vi "ThermalCam.vi"() -> ()   [LabVIEW 2024, in "ThermalCam ISGPlugin.lvlib"]
uses:
  ThermalCam ISGPlugin.lvlib
  CTI/Identity.ctl
  <vilib>/Plug-In SDKs/InstrumentStudio/Plugin Events Enum.ctl
  CTI/GPIO Pull.ctl
  1e6ec9c9-fb05-4fd0-b05f-9caec19ae962.vi
  8524c294-126d-4a78-a4f4-5e8209367d85.vi
  7e432e81-cfec-40ee-91ac-c41f46aea1a5.vi
  81a0c2b0-cfce-4e0a-bc55-b9605872672a.vi
  913d5d43-3022-4ea6-842c-e3943c591263.vi
  <extravilib>/ChannelInstances/Tag-bool/Instantiate.vi
  <extravilib>/ChannelInstances/Tag-bool/EndpointRead.vi
  <extravilib>/ChannelInstances/Tag-bool/Endpoint.vi
  <vilib>/gmath/interp.llb/Interpolate 2D (2d X,Y).vi
  CTI/Session/Session.lvclass
  <vilib>/gmath/NI_Gmath.lvlib
  <vilib>/ptbypt/NI_PtbyPt.lvlib
  <extravilib>/ChannelInstances/Tag-bool.lvlib
  CTI/VisaComms/VisaComms.lvclass
  CTI/CTI.lvlib
  <vilib>/Plug-In SDKs/InstrumentStudio/Plugin Session.lvclass
  <vilib>/Plug-In SDKs/InstrumentStudio/InstrumentStudio Plugin SDK.lvlib
panel:
  out "error out 2":errorcluster
  in  "Session Id":u64
  out "Interpolated Frame":dbl[][](graph)
  out "Unprocessed Pixels":dbl[][](graph)
  out "Processing Performance":dbl(graph)=0.0211100999986229
  out "Color Box":u32(colorbox)
  in  "Map selector":T1(ring)=enum."rainbow"
  in  "Pause":bool
  in  "Run Stop":bool
  in  "MICRO-CONTROLLER COM PORT":refnum<visa-resource-name>
  in  "SMOOTHING TYPE":i32(ring)=3 items=["nearest", "bilinear", "bicubic", "bicubic spline"]
  in  "TEMPERATURE RANGE":dbl=12.0
  in  "Interpolate":bool=TRUE
  in  "Max hold":bool
  in  "COMPRESSION":dbl=3.0
  in  "Auto Z Scale":bool=TRUE
  out "AVERAGE MAX":dbl=82.15301832388433 format="%.1f"
  out "Current Max":dbl=82.15301832388433 format="%.1f"
  in  "SMOOTHING ALPHA":dbl=0.4 min=0.0 max=1.0 step=0.05 format="%#_13g"
  out "ON-BOARD TEMP":dbl
  out "FRAME COUNT":i32
  out "Identity 2":T2
  out "error out":errorcluster
  # "ADVANCED PRESENCE SENSOR"
  # "RP2040 + AMG8833 + LabVIEW CTI"
  # "DUT Control Settings"
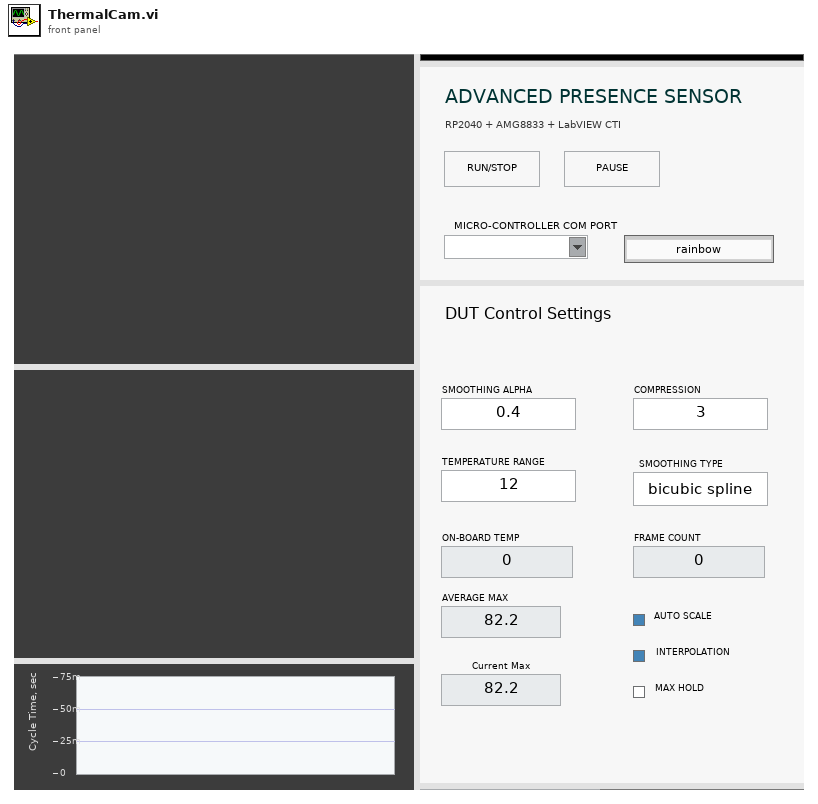
[diagram p1: front panel]
types:
  T1 = enum16{"fire", "rainbow", "grey", "inverse grey", "ice", "original"}
  T2 = typedef "CTI.lvlib/Identity.ctl" = cluster{"Vendor":string, "Model":string, "Serial":string, "Version":string}
  T3 = typedef "InstrumentStudio Plugin SDK.lvlib/Plugin Events Enum.ctl" = enum32{"Shutdown", "Project Saved", "Stop All Outputs", "Generic Message", "Active Pin Map Changed", "Selected Sites Changed"}
  T4 = typedef "Tag-bool.lvlib/))Channel.ctl" = refnum<queue>
  T5 = typedef "CTI.lvlib/GPIO Pull.ctl" = enum16{"None", "Up", "Down", "Both"}
  T6 = typedef "InstrumentStudio Plugin SDK.lvlib/Event Registration Refnum.ctl" = refnum<event-registration>
  T7 = enum16{"No Scaling", "Scale All Objects", "Scale Single Object"}
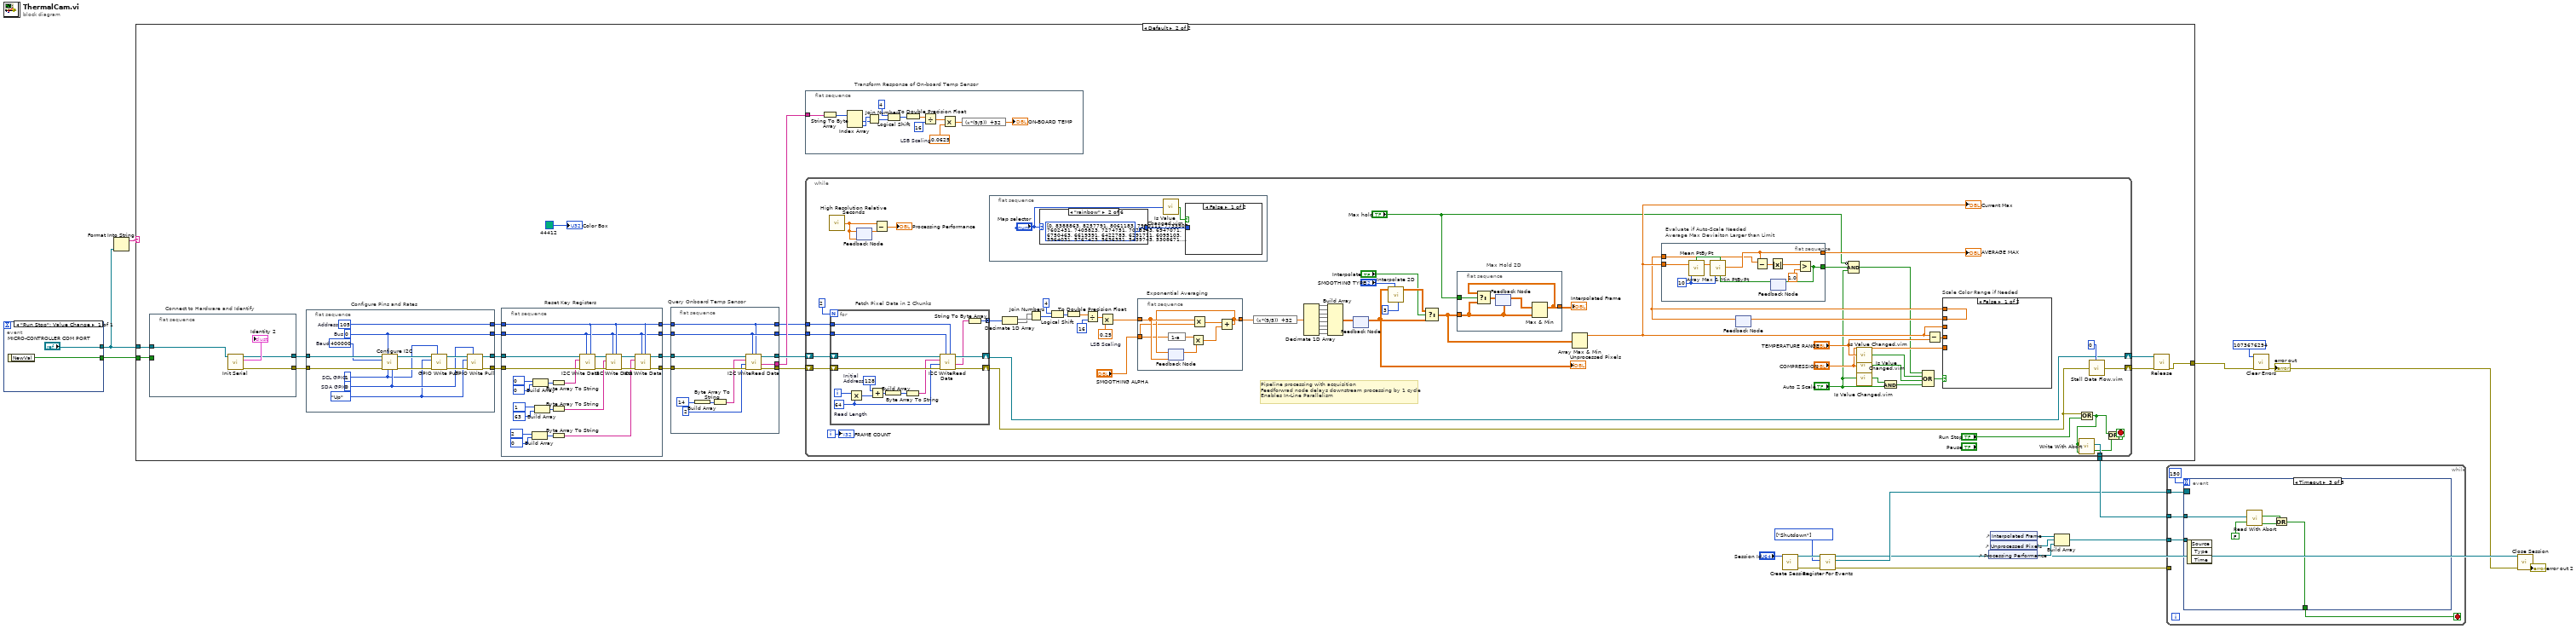
[diagram p0: block diagram]
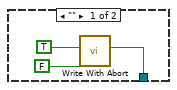
[diagram p2: hidden frame]
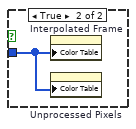
[diagram p3: hidden frame]
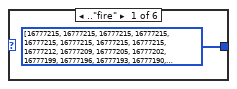
[diagram p4: hidden frame]
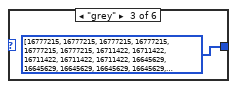
[diagram p5: hidden frame]
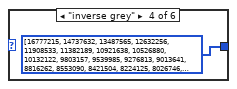
[diagram p6: hidden frame]
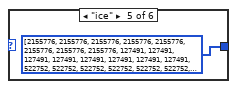
[diagram p7: hidden frame]
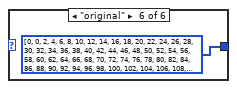
[diagram p8: hidden frame]
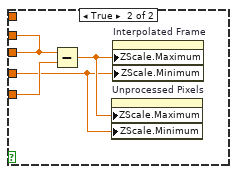
[diagram p9: hidden frame]
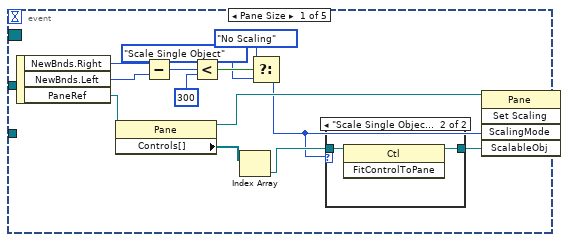
[diagram p10: hidden frame]
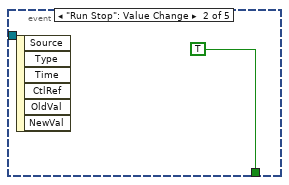
[diagram p12: hidden frame]
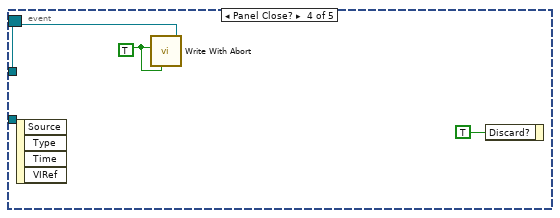
[diagram p13: hidden frame]
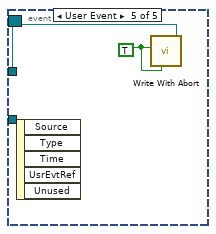
[diagram p14: hidden frame]
diagram:
  w10 = T3[] [enum."Shutdown"] items=["Shutdown", "Project Saved", "Stop All Outputs", "Generic Message", "Active Pin Map Changed", "Selected Sites Changed"] ("Events To Register")
  n1 = event shown="[0] \"Run Stop\": Value Change" {
    selector: _ -> [_]
    dyn-events: _ -> [_]
    timeout: _ -> [_]
    tunnel: [w21] -> w4
    tunnel: ["MICRO-CONTROLLER COM PORT"] -> w3
    event "Run Stop": Value Change {
      n2 = event-data() -> ("NewVal"=w21:bool)  [unwired: 1 in]
    }
  }
  n3 = Format Into String(w3) -> (resulting string=w2:string)  [unwired: 3 in, 1 out]
  n4 = case shown="Default" w2 {
    tunnel: [w24 w31] -> w14
    tunnel: w4 -> [_ w29]
    tunnel: w3 -> [_ w28]
    tunnel: [_ w25] -> w1
    frame "" {
      n5 = call <extravilib>:"Write With Abort.vi"("abort"=FALSE, "element"=TRUE) -> ("channel"=w24:T4)  [unwired: 7 in, 2 out]
    }
    frame Default {
      n6 = flat-sequence "Connect to Hardware and Identify" {
        tunnel: [w109] -> w46
        tunnel: [w108] -> w45
        tunnel: w29 -> [_]
        tunnel: w28 -> [w107]
        frame #0 {
          n7 = call "Init Serial.vi"("VISA resource name in"=w107) -> ("error out"=w108:errorcluster, "Identity"=→"Identity 2":T2, "Session"=w109:refnum<class "Session.lvclass">)  [unwired: 8 in]
        }
      }
      n8 = flat-sequence "Configure Pins and Rates" {
        tunnel: w46 -> [w106]
        tunnel: w45 -> [w105]
        tunnel: [w99] -> w44
        tunnel: [w98] -> w43
        tunnel: [w97] -> w38
        tunnel: [w96] -> w37
        frame #0 {
          w93 = GPIO_Pull."Up" ("GPIO Pull")
          w96 = u8 105  # Address
          w97 = u8 0  # Bus
          w94 = 1  # SCL GPIO
          w95 = 0  # SDA GPIO
          w104 = u32 400000  # Baud
          n9 = call "Configure I2C.vi"("SDA GPIO"=w95, "SCL GPIO"=w94, "I2C #"=w97, "error in (no error)"=w105, "Baud"=w104, "Session in"=w106) -> ("error out"=w102:errorcluster, "Session out"=w103:refnum<class "Session.lvclass">)  [unwired: 4 in]
          n10 = call "GPIO Write Pull.vi"("GPIO #"=w94, "error in (no error)"=w102, "GPIO Pull"=w93, "Session in"=w103) -> ("error out"=w100:errorcluster, "Session out"=w101:refnum<class "Session.lvclass">)  [unwired: 6 in]
          n11 = call "GPIO Write Pull.vi"("GPIO #"=w95, "error in (no error)"=w100, "GPIO Pull"=w93, "Session in"=w101) -> ("error out"=w99:errorcluster, "Session out"=w98:refnum<class "Session.lvclass">)  [unwired: 6 in]
        }
      }
      n12 = flat-sequence "Reset Key Registers" {
        tunnel: w44 -> [w92]
        tunnel: w43 -> [w91]
        tunnel: [w79] -> w42
        tunnel: [w73] -> w40
        tunnel: w38 -> [w71]
        tunnel: w37 -> [w72]
        tunnel: [w72] -> w35
        tunnel: [w71] -> w34
        frame #0 {
          n13 = Build Array(u8 2 ("Address"), u8 0 ("Address")) -> (w75:u8[])
          n14 = Build Array(u8 0 ("Address"), u8 0 ("Address")) -> (w87:u8[])
          n15 = Build Array(u8 1 ("Address"), u8 63 ("Address")) -> (w83:u8[])
          n16 = Byte Array To String(unsigned byte array=w87) -> (string=w90:string)
          n17 = Byte Array To String(unsigned byte array=w83) -> (string=w80:string)
          n18 = Byte Array To String(unsigned byte array=w75) -> (string=w74:string)
          n19 = call "I2C Write Data.vi"("Address"=w72, "I2C #"=w71, "error in (no error)"=w92, "Data"=w90, "Session in"=w91) -> ("error out"=w86:errorcluster, "Session out"=w84:refnum<class "Session.lvclass">)  [unwired: 5 in]
          n20 = call "I2C Write Data.vi"("Address"=w72, "I2C #"=w71, "error in (no error)"=w86, "Data"=w80, "Session in"=w84) -> ("error out"=w85:errorcluster, "Session out"=w78:refnum<class "Session.lvclass">)  [unwired: 5 in]
          n21 = call "I2C Write Data.vi"("Address"=w72, "I2C #"=w71, "error in (no error)"=w85, "Data"=w74, "Session in"=w78) -> ("error out"=w79:errorcluster, "Session out"=w73:refnum<class "Session.lvclass">)  [unwired: 5 in]
        }
      }
      n22 = flat-sequence "Query Onboard Temp Sensor" {
        tunnel: w42 -> [w57]
        tunnel: [w56] -> w41
        tunnel: w40 -> [w55]
        tunnel: [w54] -> w39
        tunnel: w34 -> [w48]
        tunnel: w35 -> [w47]
        tunnel: [w50] -> w36
        tunnel: [w48] -> w33
        tunnel: [w47] -> w32
        frame #0 {
          n23 = Build Array(u8 14 ("Address")) -> (w52:u8[])
          n24 = Byte Array To String(unsigned byte array=w52) -> (string=w51:string)
          n25 = call "I2C WriteRead Data.vi"("Address"=w47, "I2C #"=w48, "error in (no error)"=w57, "Len"=u8 2 ("Read Len"), "Write Data"=w51, "Session in"=w55) -> ("error out"=w56:errorcluster, "Read Data"=w50:string, "Session out"=w54:refnum<class "Session.lvclass">)  [unwired: 3 in]
        }
      }
      n26 = while {
        tunnel: w33 -> [w161]
        tunnel: w32 -> [w160]
        shift-right: [w117] -> w27
        shift-left: w41 -> [w163]
        shift-right: [w111] -> w26
        shift-left: w39 -> [w162]
        tunnel: [w116] -> w31
        i -> [w159]
        stop <- w114 stop-if-true
        w147 = 0.25  # LSB Scaling
        # "Pipeline processing with acquisition\nFeedforwrad node delays downstream processing by 1 cycle\nEnables In-Line Parallelism"
        n27 = call <vilib>:"High Resolution Relative Seconds.vi"() -> ("relative seconds"=w151:dbl)
        n28 = for "Fetch Pixel Data in 2 Chunks" {
          N: 2 -> [_]
          shift-right: [w217] -> w124
          shift-left: w163 -> [w218]
          shift-right: [w216] -> w111
          shift-left: w162 -> [w219]
          tunnel: w161 -> [w215]
          tunnel: w160 -> [w214]
          tunnel: [w220] -> w174 mode=concatenating
          i -> [w209]
          w210 = u8 64  # Read Length
          w211 = u8 128  # Initial Address
          n29 = Multiply(x=w209, y=w210) -> (x*y=w207:i32)
          n30 = Add(x=w211, y=w207) -> (x+y=w208:i32)
          n31 = Build Array(w208) -> (w221:i32[])
          n32 = Byte Array To String(unsigned byte array=w221) -> (string=w213:string)
          n33 = call "I2C WriteRead Data.vi"("Address"=w214, "I2C #"=w215, "error in (no error)"=w218, "Len"=w210, "Write Data"=w213, "Session in"=w219) -> ("error out"=w217:errorcluster, "Read Data"=w212:string, "Session out"=w216:refnum<class "Session.lvclass">)  [unwired: 3 in]
          n34 = String To Byte Array(string=w212) -> (unsigned byte array=w220:u8[])
        }
        n35 = feedback-in #1(w151) -> ()
        n36 = feedback #1(w151) -> (w150:dbl)
        n37 = Subtract(x=w151, y=w150) -> (x-y=→"Processing Performance":dbl)
        n38 = flat-sequence {
          frame #0 {
            n39 = case shown="\"rainbow\"" "Map selector" {
              tunnel: [u32[] [16777215, 16777215, 16777215, 16777215, 16777215, 16777215, 16777215, 16777215, 16777212, 16777209, 16777205, 16777202, 16777199, 16777196, 16777193, 16777190, 16777186, 16777183, 16777180, 16777177, 16777174, 16777170, 16777167, 16777164, 16777161, 16777158, 16777154, 16777151, 16777148, 16777145, 16777142, 16777139, 16777135, 16777132, 16777129, 16777126, 16777123, 16777119, 16777116, 16777113, 16777110, 16777107, 16777103, 16777100, 16777097, 16777094, 16777091, 16777088, 16777084, 16777081, 16777078, 16777075, 16777072, 16777068, 16777065, 16777062, 16777059, 16777056, 16777052, 16777049, 16777046, 16777043, 16777040, 16777037, 16777033, 16777030, 16777027, 16777024, 16777021, 16777017, 16777014, 16777011, 16777008, 16777005, 16777001, 16776998, 16776995, 16776992, 16776989, 16776986, 16776982, 16776979, 16776976, 16776973, 16776970, 16776966, 16776963, 16776960, 16776192, 16775424, 16774400, 16773632, 16772864, 16772096, 16771328, 16770560, 16769536, 16768768, 16768000, 16767232, 16766464, 16765440, 16764672, 16763904, 16763136, 16762368, 16761344, 16760576, 16759808, 16759040, 16758272, 16757504, 16756480, 16755712, 16754944, 16754176, 16753408, 16752384, 16751616, 16750848, 16750080, 16749312, 16748288, 16747520, 16746752, 16745984, 16745216, 16744448, 16743424, 16742656, 16741888, 16741120, 16740352, 16739328, 16738560, 16737792, 16737024, 16736256, 16735232, 16734464, 16733696, 16732928, 16732160, 16731392, 16730368, 16729600, 16728832, 16728064, 16727296, 16726272, 16725504, 16724736, 16723968, 16723200, 16722176, 16721408, 16720640, 16719872, 16719104, 16718336, 16717312, 16716544, 16715776, 16715008, 16714240, 16713216, 16712448, 16711680, 16515072, 16318464, 16056320, 15859712, 15663104, 15466496, 15269888, 15073280, 14811136, 14614528, 14417920, 14221312, 14024704, 13762560, 13565952, 13369344, 13172736, 12976128, 12713984, 12517376, 12320768, 12124160, 11927552, 11730944, 11468800, 11272192, 11075584, 10878976, 10682368, 10420224, 10223616, 10027008, 9830400, 9633792, 9371648, 9175040, 8978432, 8781824, 8585216, 8388608, 8126464, 7929856, 7733248, 7536640, 7340032, 7077888, 6881280, 6684672, 6488064, 6291456, 6029312, 5832704, 5636096, 5439488, 5242880, 5046272, 4784128, 4587520, 4390912, 4194304, 3997696, 3735552, 3538944, 3342336, 3145728, 2949120, 2686976, 2490368, 2293760, 2097152, 1900544, 1703936, 1441792, 1245184, 1048576, 851968, 655360, 393216, 196608, 65793, 65793, 65793, 65793, 65793, 65793, 65793, 65793, 0] ("256 fire") u32[] [0, 8388863, 8257791, 8061183, 7930111, 7733503, 7602431, 7405823, 7274751, 7078143, 6947071, 6750463, 6619391, 6422783, 6291711, 6095103, 5964031, 5767423, 5636351, 5439743, 5308671, 5112063, 4980991, 4784383, 4653311, 4456703, 4325631, 4129023, 3932415, 3801343, 3604735, 3473663, 3277055, 3145983, 2949375, 2818303, 2621695, 2490623, 2294015, 2162943, 1966335, 1835263, 1638655, 1507583, 1310975, 1179903, 983295, 852223, 655615, 524543, 327935, 196863, 511, 1791, 3071, 4351, 5631, 6911, 8191, 9471, 10751, 12031, 13311, 14591, 15871, 17151, 18431, 19711, 20991, 22271, 23551, 24831, 26111, 27391, 28671, 29951, 31231, 32511, 33791, 35071, 36351, 37631, 38911, 40191, 41471, 42751, 44031, 45311, 46591, 47871, 49151, 50431, 51711, 52991, 54271, 55551, 56831, 58111, 59391, 60671, 61951, 63231, 64511, 65532, 65527, 65522, 65517, 65512, 65507, 65502, 65497, 65492, 65487, 65482, 65477, 65472, 65467, 65462, 65457, 65452, 65447, 65442, 65437, 65432, 65427, 65422, 65417, 65412, 65407, 65402, 65397, 65392, 65387, 65382, 65377, 65372, 65367, 65362, 65357, 65352, 65347, 65342, 65337, 65332, 65327, 65322, 65317, 65312, 65307, 65302, 65297, 65292, 65287, 65282, 261888, 589568, 917248, 1244928, 1572608, 1900288, 2227968, 2555648, 2883328, 3211008, 3538688, 3866368, 4194048, 4521728, 4849408, 5177088, 5504768, 5832448, 6160128, 6487808, 6815488, 7143168, 7470848, 7798528, 8126208, 8453888, 8781568, 9109248, 9436928, 9764608, 10092288, 10419968, 10747648, 11075328, 11403008, 11730688, 12058368, 12386048, 12713728, 13041408, 13369088, 13696768, 14024448, 14352128, 14679808, 15007488, 15335168, 15662848, 15990528, 16318208, 16645888, 16775936, 16774656, 16773376, 16772096, 16770816, 16769536, 16768256, 16766976, 16765696, 16764416, 16763136, 16761856, 16760576, 16759296, 16758016, 16756736, 16755456, 16754176, 16752896, 16751616, 16750336, 16749056, 16747776, 16746496, 16745216, 16743936, 16742656, 16741376, 16740096, 16738816, 16737536, 16736256, 16734976, 16733696, 16732416, 16731136, 16729856, 16728576, 16727296, 16726016, 16724736, 16723456, 16722176, 16720896, 16719616, 16718336, 16717056, 16715776, 16714496, 16713216, 16711680] ("rainbow") u32[] [16777215, 16777215, 16777215, 16777215, 16777215, 16777215, 16711422, 16711422, 16711422, 16711422, 16711422, 16645629, 16645629, 16645629, 16645629, 16645629, 16645629, 16579836, 16579836, 16579836, 16579836, 16579836, 16514043, 16514043, 16514043, 16514043, 16514043, 16448250, 16448250, 16448250, 16448250, 16448250, 16316664, 16382457, 16382457, 16382457, 16382457, 16316664, 16316664, 16316664, 16316664, 16250871, 16250871, 16250871, 16250871, 16250871, 16185078, 16185078, 16185078, 16185078, 16119285, 16119285, 16119285, 16119285, 16119285, 16053492, 16053492, 16053492, 16053492, 15987699, 15987699, 15987699, 15987699, 15921906, 15987699, 15921906, 15921906, 15856113, 15856113, 15856113, 15856113, 15856113, 15790320, 15790320, 15790320, 15724527, 15724527, 15724527, 15724527, 15658734, 15658734, 15658734, 15658734, 15592941, 15592941, 15592941, 15592941, 15527148, 15527148, 15527148, 15461355, 15461355, 15461355, 15461355, 15395562, 15395562, 15395562, 15395562, 15329769, 15329769, 15329769, 15263976, 15263976, 15263976, 15198183, 15198183, 15198183, 15198183, 15132390, 15132390, 15132390, 15066597, 15066597, 15066597, 15000804, 15000804, 15000804, 14935011, 14935011, 14935011, 14869218, 14869218, 14869218, 14803425, 14803425, 14803425, 14737632, 14737632, 14671839, 14671839, 14671839, 14606046, 14606046, 14606046, 14540253, 14540253, 14540253, 14474460, 14474460, 14408667, 14408667, 14408667, 14342874, 14342874, 14277081, 14277081, 14277081, 14211288, 14211288, 14145495, 14145495, 14079702, 14079702, 14013909, 14013909, 14013909, 13948116, 13948116, 13882323, 13882323, 13816530, 13816530, 13750737, 13750737, 13684944, 13684944, 13619151, 13619151, 13553358, 13553358, 13487565, 13487565, 13421772, 13421772, 13355979, 13290186, 13290186, 13224393, 13224393, 13158600, 13092807, 13092807, 13027014, 13027014, 12961221, 12895428, 12895428, 12829635, 12763842, 12763842, 12698049, 12632256, 12566463, 12566463, 12500670, 12434877, 12434877, 12369084, 12303291, 12237498, 12171705, 12171705, 12105912, 12040119, 11974326, 11908533, 11842740, 11776947, 11711154, 11645361, 11579568, 11513775, 11447982, 11382189, 11316396, 11250603, 11184810, 11119017, 10987431, 10921638, 10855845, 10790052, 10658466, 10592673, 10461087, 10395294, 10329501, 10197915, 10066329, 10000536, 9868950, 9737364, 9605778, 9474192, 9342606, 9211020, 9079434, 8882055, 8750469, 8553090, 8421504, 8224125, 7960953, 7763574, 7500402, 7237230, 6974058, 6645093, 6316128, 5855577, 5395026, 4868682, 4210752, 3289650, 2105376, 0] ("256 log up") u32[] [16777215, 14737632, 13487565, 12632256, 11908533, 11382189, 10921638, 10526880, 10132122, 9803157, 9539985, 9276813, 9013641, 8816262, 8553090, 8421504, 8224125, 8026746, 7895160, 7697781, 7566195, 7434609, 7303023, 7171437, 7039851, 6908265, 6776679, 6710886, 6579300, 6447714, 6381921, 6316128, 6184542, 6118749, 5987163, 5921370, 5855577, 5789784, 5658198, 5592405, 5526612, 5460819, 5395026, 5329233, 5263440, 5197647, 5131854, 5066061, 5000268, 4934475, 4868682, 4802889, 4737096, 4671303, 4605510, 4605510, 4539717, 4473924, 4408131, 4342338, 4342338, 4276545, 4210752, 4210752, 4144959, 4079166, 4013373, 4013373, 3947580, 3881787, 3881787, 3815994, 3750201, 3750201, 3684408, 3684408, 3618615, 3552822, 3552822, 3487029, 3487029, 3421236, 3421236, 3355443, 3289650, 3289650, 3223857, 3223857, 3158064, 3158064, 3092271, 3092271, 3026478, 3026478, 2960685, 2960685, 2894892, 2894892, 2829099, 2829099, 2763306, 2763306, 2763306, 2697513, 2697513, 2631720, 2631720, 2565927, 2565927, 2500134, 2500134, 2500134, 2434341, 2434341, 2368548, 2368548, 2368548, 2302755, 2302755, 2236962, 2236962, 2236962, 2171169, 2171169, 2171169, 2105376, 2105376, 2105376, 2039583, 2039583, 1973790, 1973790, 1973790, 1907997, 1907997, 1907997, 1842204, 1842204, 1842204, 1776411, 1776411, 1776411, 1710618, 1710618, 1710618, 1644825, 1644825, 1644825, 1579032, 1579032, 1579032, 1579032, 1513239, 1513239, 1513239, 1447446, 1447446, 1447446, 1381653, 1381653, 1381653, 1381653, 1315860, 1315860, 1315860, 1315860, 1250067, 1250067, 1250067, 1184274, 1184274, 1184274, 1184274, 1118481, 1118481, 1118481, 1118481, 1052688, 1052688, 1052688, 1052688, 986895, 986895, 986895, 921102, 921102, 921102, 921102, 921102, 855309, 855309, 855309, 855309, 789516, 789516, 789516, 789516, 723723, 723723, 723723, 723723, 657930, 657930, 657930, 657930, 657930, 592137, 592137, 592137, 592137, 526344, 526344, 526344, 526344, 526344, 460551, 460551, 460551, 460551, 460551, 394758, 394758, 394758, 394758, 328965, 328965, 328965, 328965, 328965, 263172, 263172, 263172, 263172, 263172, 197379, 197379, 197379, 197379, 197379, 131586, 131586, 131586, 131586, 131586, 131586, 65793, 65793, 65793, 65793, 65793, 0, 0, 0, 0, 0, 0] ("256 log down") u32[] [2155776, 2155776, 2155776, 2155776, 2155776, 2155776, 2155776, 2155776, 127491, 127491, 127491, 127491, 127491, 127491, 127491, 127491, 522752, 522752, 522752, 522752, 522752, 522752, 522752, 522752, 64018, 64018, 64018, 64018, 64018, 64018, 64018, 64018, 63778, 63778, 63778, 63778, 63778, 63778, 63778, 63778, 63790, 63790, 63790, 63790, 63790, 63790, 63790, 63790, 63797, 63797, 63797, 63797, 63797, 63797, 63797, 63797, 63807, 63807, 63807, 63807, 63807, 63807, 63807, 63807, 64068, 64068, 64068, 64068, 64068, 64068, 64068, 64068, 63828, 63828, 63828, 63828, 63828, 63828, 63828, 63828, 63833, 63833, 63833, 63833, 63833, 63833, 63833, 63833, 63836, 63836, 63836, 63836, 63836, 63836, 63836, 63836, 63836, 63836, 63836, 63836, 63836, 63836, 63836, 63836, 61790, 61790, 61790, 61790, 61790, 61790, 61790, 61790, 58464, 58464, 58464, 58464, 58464, 58464, 58464, 58464, 55387, 55387, 55387, 55387, 55387, 55387, 55387, 55387, 51286, 51286, 51286, 51286, 51286, 51286, 51286, 51286, 47440, 47440, 47440, 47440, 47440, 47440, 47440, 47440, 40284, 40284, 40284, 40284, 40284, 40284, 40284, 40284, 34154, 34154, 34154, 34154, 34154, 34154, 34154, 34154, 28540, 28540, 28540, 28540, 28540, 28540, 28540, 28540, 20113, 20113, 20113, 20113, 20113, 20113, 20113, 20113, 12193, 12193, 12193, 12193, 12193, 12193, 12193, 12193, 12714, 12714, 12714, 12714, 12714, 12714, 12714, 12714, 7351, 7351, 7351, 7351, 7351, 7351, 7351, 7351, 4800, 4800, 4800, 4800, 4800, 4800, 4800, 4800, 195, 195, 195, 195, 195, 195, 195, 195, 189, 189, 189, 189, 189, 189, 189, 189, 183, 183, 183, 183, 183, 183, 183, 183, 175, 175, 175, 175, 175, 175, 175, 175, 164, 164, 164, 164, 164, 164, 164, 164, 155, 155, 155, 155, 155, 155, 155, 155] ("32 ice") u32[] [0, 0, 2, 4, 6, 8, 10, 12, 14, 16, 18, 20, 22, 24, 26, 28, 30, 32, 34, 36, 38, 40, 42, 44, 46, 48, 50, 52, 54, 56, 58, 60, 62, 64, 66, 68, 70, 72, 74, 76, 78, 80, 82, 84, 86, 88, 90, 92, 94, 96, 98, 100, 102, 104, 106, 108, 110, 112, 114, 116, 118, 120, 122, 124, 126, 128, 130, 132, 134, 136, 138, 140, 142, 144, 146, 148, 150, 152, 154, 156, 158, 160, 162, 164, 166, 168, 170, 172, 174, 176, 178, 180, 182, 184, 186, 188, 190, 192, 194, 196, 198, 200, 202, 204, 206, 208, 210, 212, 214, 216, 218, 220, 222, 224, 226, 228, 230, 232, 234, 236, 238, 240, 242, 244, 246, 248, 250, 252, 255, 131839, 263423, 395007, 526591, 658175, 789759, 921343, 1052927, 1184511, 1316095, 1447679, 1579263, 1710847, 1842431, 1974015, 2105599, 2237183, 2368767, 2500351, 2631935, 2763519, 2895103, 3026687, 3158271, 3289855, 3421439, 3553023, 3684607, 3816191, 3947775, 4079359, 4210943, 4342527, 4474111, 4605695, 4737279, 4868863, 5000447, 5132031, 5263615, 5395199, 5526783, 5658367, 5789951, 5921535, 6053119, 6184703, 6316287, 6447871, 6579455, 6711039, 6842623, 6974207, 7105791, 7237375, 7368959, 7500543, 7632127, 7763711, 7895295, 8026879, 8158463, 8290047, 8421631, 8553215, 8684799, 8816383, 8947967, 9079551, 9211135, 9342719, 9474303, 9605887, 9737471, 9869055, 10000639, 10132223, 10263807, 10395391, 10526975, 10658559, 10790143, 10921727, 11053311, 11184895, 11316479, 11448063, 11579647, 11711231, 11842815, 11974399, 12105983, 12237567, 12369151, 12500735, 12632319, 12763903, 12895487, 13027071, 13158655, 13290239, 13421823, 13553407, 13684991, 13816575, 13948159, 14079743, 14211327, 14342911, 14474495, 14606079, 14737663, 14869247, 15000831, 15132415, 15263999, 15395583, 15527167, 15658751, 15790335, 15921919, 16053503, 16185087, 16316671, 16448255, 16579839, 16777215] ("original")] -> w192
              frame .."fire" {
              }
              frame "rainbow" {
              }
              frame "grey" {
              }
              frame "inverse grey" {
              }
              frame "ice" {
              }
              frame "original" {
              }
            }
            n40 = call "Is Value Changed.vim"("value"="Map selector") -> ("changed or first call?"=w190:bool)
            n41 = case shown="False" w190 {
              tunnel: w192 -> [_ w193]
              frame False {
              }
              frame True {
                n42 = property on="Interpolated Frame" class="IntGraph (strict)"("Color Table"=w193) -> ()  [unwired: 2 in, 2 out]
                n43 = property on="Unprocessed Pixels" class="IntGraph (strict)"("Color Table"=w193) -> ()  [unwired: 2 in, 2 out]
              }
            }
          }
        }
        n44 = Decimate 1D Array(w174) -> (w173:u8[], w172:u8[])
        n45 = Join Numbers(hi=w172, lo=w173) -> ((hi.lo)=w154:u16[])
        n46 = Logical Shift(y=i16 4, x=w154) -> (x << y=w157:u16[])
        n47 = To Double Precision Float(number=w157) -> (double precision float=w156:dbl[])
        n48 = Divide(x=w156, y=i16 16) -> (x/y=w153:dbl[])
        n49 = Multiply(x=w153, y=w147) -> (x*y=w145:dbl[])
        n50 = flat-sequence "Exponential Averaging" {
          tunnel: w145 -> [w202]
          tunnel: [w201] -> w144
          tunnel: "SMOOTHING ALPHA" -> [w200]
          frame #0 {
            n51 = expression code="1-a"(w200) -> (w205:dbl)
            n52 = feedback #2(w202) -> (w203:dbl[])
            n53 = Multiply(x=w205, y=w203) -> (x*y=w204:dbl[])
            n54 = Multiply(x=w202, y=w200) -> (x*y=w206:dbl[])
            n55 = Add(x=w206, y=w204) -> (x+y=w201:dbl[])
            n56 = feedback-in #2(w201) -> ()
          }
        }
        n57 = expression code="(x*(9/5))  +32"(w144) -> (w152:dbl[])
        n58 = Decimate 1D Array(w152) -> (w164:dbl[], w165:dbl[], w166:dbl[], w167:dbl[], w168:dbl[], w169:dbl[], w170:dbl[], w171:dbl[])
        n59 = Build Array(w164, w165, w166, w167, w168, w169, w170, w171) -> (w127:dbl[][])
        n60 = feedback-in #3(w127) -> ()
        n61 = feedback #3() -> (w123:dbl[][])  [unwired: 1 in]
        "Unprocessed Pixels" <- w123
        n62 = call-poly <vilib>:"Interpolate 2D.vi"("ntimes"=3, "method"="SMOOTHING TYPE", "Z"=w123) -> ("zi"=w137:dbl[][])  [unwired: 5 in, 3 out]
        n63 = Select(t=w137, s="Interpolate", f=w123) -> (s? t:f=w136:dbl[][])
        n64 = flat-sequence "Max Hold 2D" {
          tunnel: [w178] -> w138
          tunnel: w136 -> [w176]
          tunnel: "Max hold" -> [w175]
          frame #0 {
            n65 = feedback #4(w176) -> (w179:dbl[][])
            n66 = Max & Min(x=w179, y=w176) -> (max(x,y)=w178:dbl[][])  [unwired: 1 out]
            n67 = Select(t=w178, s=w175, f=w176) -> (s? t:f=w177:dbl[][])
            n68 = feedback-in #4(w177) -> ()
          }
        }
        n69 = Array Max & Min(array=w136) -> (max value=w139:dbl)  [unwired: 3 out]
        "Current Max" <- w139
        n70 = flat-sequence "Evaluate if Auto-Scale Needed\nAverage Max Deviaiton Larger than Limit" {
          tunnel: [w183] -> w141
          tunnel: w139 -> [w182]
          tunnel: w125 -> [w181]
          tunnel: [w180] -> w130
          frame #0 {
            w185 = 10 ("sample length")
            n71 = feedback #5() -> (w184:bool)  [unwired: 1 in]
            n72 = call <vilib>:"Mean PtByPt.vi"("x"=w182, "sample length"=w185, "initialize"=w184) -> ("mean"=w186:dbl)  [unwired: 1 in, 1 out]
            n73 = call <vilib>:"Array Max & Min PtByPt.vi"("input data point"=w186, "sample length"=w185, "initialize"=w184) -> ("max value"=w183:dbl)  [unwired: 4 out]
            n74 = Subtract(x=w181, y=w183) -> (x-y=w189:dbl)
            n75 = Absolute Value(x=w189) -> (abs(x)=w188:dbl)
            n76 = Greater?(x=w188, y=1.0) -> (0:w180:bool)
            n77 = feedback-in #5(w180) -> ()
          }
        }
        n78 = feedback #6() -> (w125:dbl)  [unwired: 1 in]
        n79 = Compound Arithmetic op=AND(invert "Max hold", w130, "Auto Z Scale") -> (w122:bool)
        n80 = call "Is Value Changed.vim"("value"="TEMPERATURE RANGE") -> ("changed or first call?"=w142:bool)
        n81 = call "Is Value Changed.vim"("value"="COMPRESSION") -> ("changed or first call?"=w133:bool)
        n82 = call "Is Value Changed.vim"("value"="Auto Z Scale") -> ("changed or first call?"=w132:bool)
        n83 = And(x=w132, y="Auto Z Scale") -> (x .and. y?=w120:bool)
        n84 = Compound Arithmetic op=OR(w122, w142, w133, w120) -> (w121:bool)
        n85 = Subtract(x=w139, y="TEMPERATURE RANGE") -> (x-y=w146:dbl)
        n86 = case "Scale Color Range if Needed" shown="False" w121 {
          tunnel: w146 -> [_ w223]
          tunnel: w139 -> [_ w226]
          tunnel: [w222 w226] -> w140
          tunnel: w125 -> [w222 _]
          tunnel: "COMPRESSION" -> [_ w225]
          frame False {
          }
          frame True {
            n87 = Subtract(x=w226, y=w225) -> (x-y=w224:dbl)
            n88 = property on="Unprocessed Pixels" class="IntGraph (strict)"("ZScale.Maximum"=w224, "ZScale.Minimum"=w223) -> ()  [unwired: 2 in, 2 out]
            n89 = property on="Interpolated Frame" class="IntGraph (strict)"("ZScale.Maximum"=w224, "ZScale.Minimum"=w223) -> ()  [unwired: 2 in, 2 out]
          }
        }
        n90 = feedback-in #6(w140) -> ()
        n91 = Compound Arithmetic op=OR(w124, "Run Stop") -> (w115:bool)
        n92 = call <extravilib>:"Write With Abort.vi"("abort"=w115, "element"=w115) -> ("channel"=w116:T4, "aborted?"=w113:bool)  [unwired: 7 in, 1 out]
        n93 = call "Stall Data Flow.vim"("value in"=w124, "milliseconds to wait"=u32 0) -> ("value out"=w117:errorcluster)  [unwired: 1 out]
        n94 = Or(x=w115, y=w113) -> (x .or. y?=w114:bool)
        "Interpolated Frame" <- w138
        "FRAME COUNT" <- w159
        "AVERAGE MAX" <- w141
      }
      n95 = flat-sequence "Transform Response of On-board Temp Sensor" {
        tunnel: w36 -> [w70]
        frame #0 {
          w58 = 0.0625  # LSB Scaling
          n96 = String To Byte Array(string=w70) -> (unsigned byte array=w69:u8[])
          n97 = Index Array(array=w69) -> (element #1=w67:u8, element #2=w68:u8)  [unwired: 2 in]
          n98 = Join Numbers(hi=w68, lo=w67) -> ((hi.lo)=w60:u16)
          n99 = Logical Shift(y=i16 4, x=w60) -> (x << y=w63:u16)
          n100 = To Double Precision Float(number=w63) -> (double precision float=w64:dbl)
          n101 = Divide(x=w64, y=i16 16) -> (x/y=w66:dbl)
          n102 = Multiply(x=w66, y=w58) -> (x*y=w59:dbl)
          n103 = expression code="(x*(9/5))  +32"(w59) -> (→"ON-BOARD TEMP":dbl)
        }
      }
      n104 = call-dynamic "Release.vi"("error in (no error)"=w27, "Session in"=w26) -> ("error out"=w25:errorcluster)  [unwired: 9 in]
      "Color Box" <- u32 44412 ("Color Box")
    }
  }
  n105 = call <vilib>:"Create Session.vi"("Session Id"="Session Id") -> ("error out"=w13:errorcluster, "Session out"=w12:refnum<class "Plugin Session.lvclass">)  [unwired: 6 in, 3 out]
  n106 = call <vilib>:"Register For Events.vi"("error in (no error)"=w13, "Events To Register"=w10, "Session in"=w12) -> ("error out"=w6:errorcluster, "Event Refnum"=w9:T6, "Session out"=w8:refnum<class "Plugin Session.lvclass">)  [unwired: 6 in]
  n107 = control-ref of="Processing Performance"() -> (w15:refnum<vi>)
  n108 = control-ref of="Interpolated Frame"() -> (w16:refnum<vi>)
  n109 = control-ref of="Unprocessed Pixels"() -> (w18:refnum<vi>)
  n110 = Build Array(w16, w18, w15) -> (w17:refnum<vi>[])
  n111 = while {
    tunnel: w17 -> [w230]
    tunnel: w14 -> [w228]
    tunnel: w9 -> [w227]
    tunnel: w6 -> [_]
    stop <- w231 stop-if-true
    n112 = event shown="[2] Timeout" {
      selector: w227 -> [_ _ _ _ _]
      dyn-events: _ -> [_ _ _ _ _]
      timeout: 150 -> [_ _ _ _ _]
      tunnel: [_ TRUE w249 _ _] -> w231
      tunnel: w230 -> [_ _ _ _ _]
      tunnel: [_ _ w251 w255 w258] -> w228
      event Pane Size {
        n113 = event-data() -> ("NewBnds.Right"=w244:i16, "NewBnds.Left"=w243:i16, "PaneRef"=w240:refnum<vi>)  [unwired: 1 in]
        n114 = property class="Pane"(reference=w240) -> (reference out=w235:refnum<vi>, "Controls[]"=w239:refnum<vi>[])  [unwired: 1 in, 1 out]
        n115 = Subtract(x=w244, y=w243) -> (x-y=w242:i16)
        n116 = Less?(x=w242, y=i16 300) -> (x < y?=w238:bool)
        n117 = Index Array(array=w239) -> (element=w234:refnum<vi>)  [unwired: 1 in]
        n118 = Select(t=T7."No Scaling" ("Scaling Mode"), s=w238, f=T7."Scale Single Object" ("Scaling Mode")) -> (s? t:f=w232:T7)
        n119 = case shown="\"Scale Single Object\"" w232 {
          tunnel: w234 -> [w245 w247]
          tunnel: [w245 w246] -> w233
          frame "No Scaling", Default {
          }
          frame "Scale Single Object" {
            n120 = invoke class="Ctl" method="FitControlToPane"(reference=w247) -> (reference out=w246:refnum<vi>)  [unwired: 2 in, 2 out]
          }
        }
        n121 = invoke class="Pane" method="Set Scaling"(reference=w235, "ScalingMode"=w232, "ScalableObj"=w233) -> ()  [unwired: 2 in, 5 out]
      }
      event "Run Stop": Value Change {
        n122 = event-data() -> ()  [unwired: 1 in, 6 out]
      }
      event Timeout {
        n123 = event-data() -> ()  [unwired: 1 in, 3 out]
        n124 = call <extravilib>:"Read With Abort.vi"("abort"=FALSE, "channel"=w251) -> ("element"=w253:bool, "aborted?"=w250:bool)  [unwired: 7 in, 1 out]
        n125 = Or(x=w253, y=w250) -> (x .or. y?=w249:bool)
      }
      event Panel Close? {
        w254 = TRUE ("element")
        n126 = event-data() -> ()  [unwired: 1 in, 4 out]
        n127 = call <extravilib>:"Write With Abort.vi"("abort"=w254, "element"=w254) -> ("channel"=w255:T4)  [unwired: 7 in, 2 out]
        n128 = event-data("Discard?"=TRUE) -> ()  [unwired: 1 in, 1 out]
      }
      event User Event {
        w257 = TRUE ("element")
        n129 = event-data() -> ()  [unwired: 1 in, 5 out]
        n130 = call <extravilib>:"Write With Abort.vi"("abort"=w257, "element"=w257) -> ("channel"=w258:T4)  [unwired: 7 in, 2 out]
      }
    }
  }
  n131 = call <vilib>:"Clear Errors.vi"("error in (no error)"=w1, "specific error code to clear (0: all)"=1073676294) -> ("error out"=w7:errorcluster)  [unwired: 4 in, 1 out]
  "error out" <- w7
  n132 = call <vilib>:"Close Session.vi"("error in (no error)"=w7, "Session in"=w8) -> ("error out"=→"error out 2":errorcluster)  [unwired: 9 in]
